vi "ErrorHandler.vi"(8 "Error In":errorcluster, 11 "MainDataIn":T1={"Image"={"image type"=0, "image depth"=32, "image"=array[640000 elements], "mask"=array[20000 elements], "colors"=[], "Rectangle"={"left"=0, "top"=0, "right"=400, "bottom"=400}}, " TmpImage"={"image type"=0, "image depth"=32, "image"=array[640000 elements], "mask"=array[20000 elements], "colors"=[], "Rectangle"={"left"=0, "top"=0, "right"=400, "bottom"=400}}, "BGColor"=15256322, "FGColor"=13283586, "DRColor"=13283586, "Picture"=bytes[500030], "Queue "=refnum, "EndGameEvent"=refnum, "AnalizeMove"=FALSE}) -> ()   [LabVIEW 2020]
uses:
  typeDef/MainDataCluster.ctl
  <vilib>/picture/picture.llb/imagedata.ctl
  typeDef/StateMachineEnum.ctl
  typeDef/EventData.ctl
  typeDef/EndType.ctl
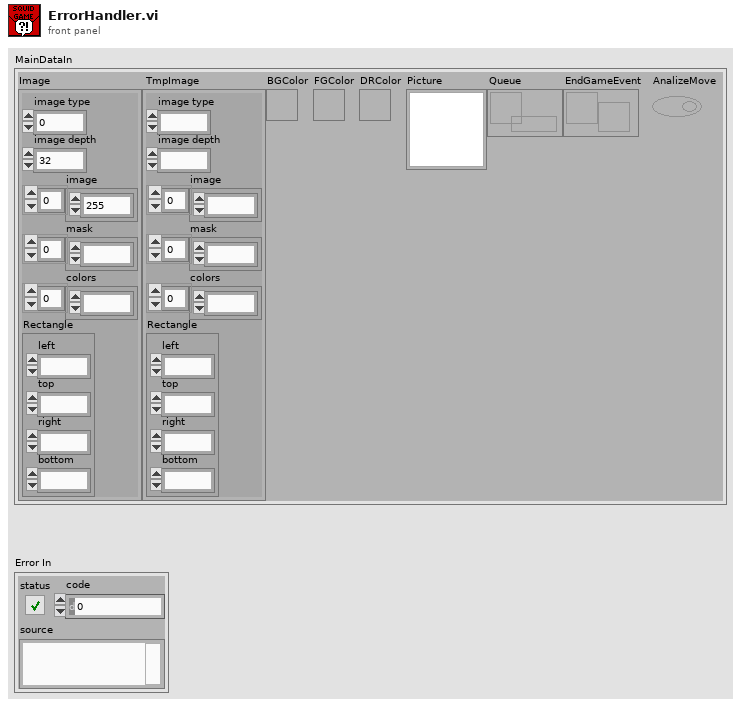
[diagram p1: front panel]
types:
  T1 = typedef "MainDataCluster.ctl" = cluster{"Image":T2, " TmpImage":T2, "BGColor":u32, "FGColor":u32, "DRColor":u32, "Picture":picture, "Queue ":refnum<queue>, "EndGameEvent":refnum<user-event>, "AnalizeMove":bool}
  T2 = typedef "imagedata.ctl" = cluster{"image type":i32, "image depth":i32, "image":u8[], "mask":u8[], "colors":u32[], "Rectangle":cluster{"left":i16, "top":i16, "right":i16, "bottom":i16}}
  T3 = typedef "EventData.ctl" = cluster{"ShowResult":bool, "EndingType":T4}
  T4 = typedef "EndType.ctl" = enum16{"Timeout", "MouseUp", "OutOfLine", "CloseLine", "UserEnd"}
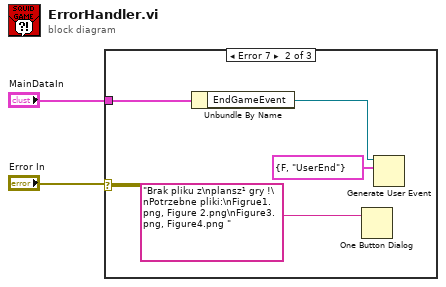
[diagram p0: block diagram]
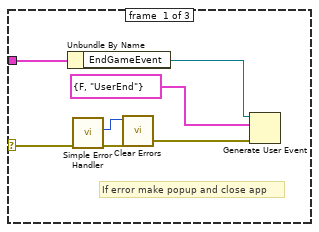
[diagram p2: hidden frame]
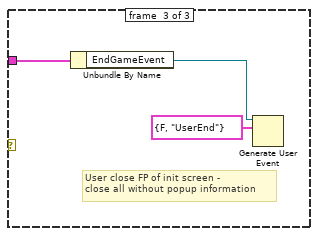
[diagram p3: hidden frame]
diagram:
  n1 = case shown="Error 7" "Error In" {
    selector: "Error In" -> [w9 _ _]
    tunnel: "MainDataIn" -> [w6 w11 w16]
    frame #0 {
      # "If error make popup and close app"
      n2 = Unbundle By Name(w6) -> ("EndGameEvent"=w8:refnum<user-event>)
      n3 = call <vilib>:"Simple Error Handler.vi"("error in (no error)"=w9) -> ("code out"=w4:i32, "error out"=w5:errorcluster)  [unwired: 4 in, 3 out]
      n4 = call <vilib>:"Clear Errors.vi"("error in (no error)"=w5, "specific error code to clear (0: all)"=w4) -> ("error out"=w3:errorcluster)  [unwired: 4 in, 1 out]
      n5 = Generate User Event(user event=w8, event data cluster=T3 {"ShowResult"=FALSE, "EndingType"=enum."UserEnd"} ("event data"), error in=w3) -> ()  [unwired: 1 in, 2 out]
    }
    frame #1 {
      n6 = Unbundle By Name(w11) -> ("EndGameEvent"=w13:refnum<user-event>)
      n7 = One Button Dialog(message="Brak pliku z\nplansz¹ gry !\nPotrzebne pliki:\nFigrue1.png, Figure 2.png\nFigure3.png, Figure4.png ") -> ()  [unwired: 1 in, 1 out]
      n8 = Generate User Event(user event=w13, event data cluster=T3 {"ShowResult"=FALSE, "EndingType"=enum."UserEnd"} ("event data")) -> ()  [unwired: 2 in, 2 out]
    }
    frame #2 {
      # "User close FP of init screen -\nclose all without popup information"
      n9 = Unbundle By Name(w16) -> ("EndGameEvent"=w15:refnum<user-event>)
      n10 = Generate User Event(user event=w15, event data cluster=T3 {"ShowResult"=FALSE, "EndingType"=enum."UserEnd"} ("event data")) -> ()  [unwired: 2 in, 2 out]
    }
  }
